vi "Get Version Information.vi"(8 "error in (no error)":errorcluster, 11 "NI_AB_API_Targetfile in":refnum<class "NI_AB_API_Targetfile.lvclass">) -> (0 "error out":errorcluster, 2 "Version Information":T1, 3 "NI_AB_API_Targetfile out":refnum<class "NI_AB_API_Targetfile.lvclass">)   [LabVIEW 2020, in "NI_AB_API_Targetfile.lvclass"]
uses:
  <vilib>/AppBuilder/AB_API/Targetfile/NI_AB_API_Targetfile.lvclass
  e:/builds/penguin/labview/branches/2020/dev/dist/vi.lib/AppBuilder/AB_API/Build/NI_AB_API_Build.lvclass
  <vilib>/AppBuilder/AB_API/common/AB_API Version Information.ctl
  <vilib>/AppBuilder/AB_Classes/TargetFile/AB_Targetfile.lvclass
  <vilib>/AppBuilder/AB_API/Targetfile/NI_AB_API_Targetfile.lvclass/NI_AB_API_Targetfile.ctl
  <vilib>/AppBuilder/AB_API/Build/NI_AB_API_Build.lvclass
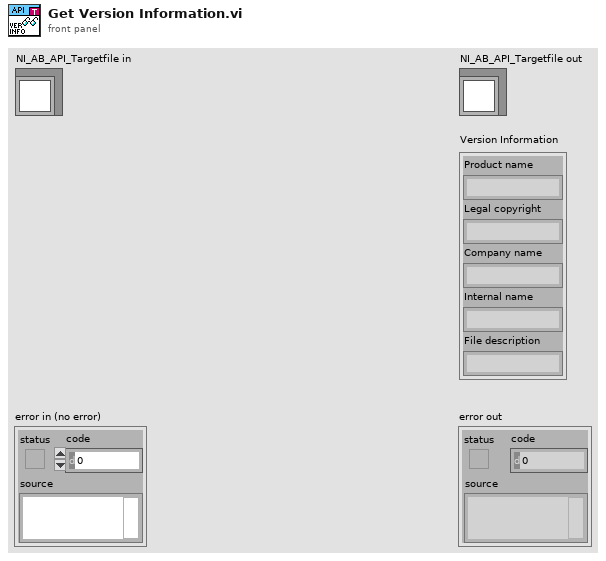
[diagram p1: front panel]
types:
  T1 = typedef "AB_API Version Information.ctl" = cluster{"Product name":string, "Legal copyright":string, "Company name":string, "Internal name":string, "File description":string}
  T2 = typedef "AB_Targetfile.ctl" = cluster{"targetfileName":string, "targetfileGUID":string, "enableDebugging":bool, "versionInfo":cluster{"productName":string, "legalCopyright":string, "companyName":string, "internalName":string, "fileDescription":string}, "eng_consolidatedTypeInfo":string, "fastFileFormat":bool, "eng_LEIFBuildData":u32, "versionIndependent":bool}
  T3 = cluster{"productName":string, "legalCopyright":string, "companyName":string, "internalName":string, "fileDescription":string}
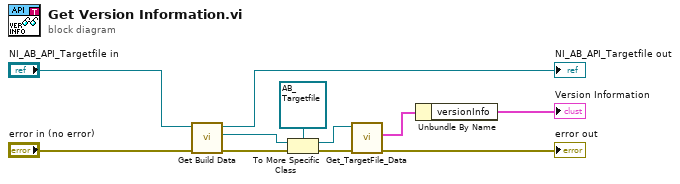
[diagram p0: block diagram]
diagram:
  n1 = call <vilib>:"Get Build Data.vi"("error in (no error)"="error in (no error)", "NI_AB_API_Build in"="NI_AB_API_Targetfile in") -> ("error out"=w6:errorcluster, "AB_Build.lvclass"=w5:refnum<class "AB_Build.lvclass">, "NI_AB_API_Build out"=→"NI_AB_API_Targetfile out":refnum<class "NI_AB_API_Targetfile.lvclass">)  [unwired: 7 in]
  n2 = To More Specific Class(target class=refnum<class "AB_Targetfile.lvclass"> refnum ("AB_Targetfile in"), reference=w5, error in=w6) -> (specific class reference=w3:refnum<class "AB_Targetfile.lvclass">, error out=w2:errorcluster)
  n3 = call <vilib>:"Get_TargetFile_Data.vi"("error in (no error)"=w2, "AB_Targetfile in"=w3) -> ("error out"=→"error out":errorcluster, "data"=w1:T2)  [unwired: 7 in, 1 out]
  n4 = Unbundle By Name(w1) -> ("versionInfo"=→"Version Information":T3)
